vi "Main Page.vi"(8 "error in (no error)":errorcluster, 11 "Node Ptr":T2 format="%.0x") -> (0 "error out":errorcluster)   [LabVIEW 2019, in "TimingDRV System Explorer.lvlib"]
uses:
  TimingDRV System Explorer.lvlib
  <vilib>/NI VeriStand/Custom Device API/Custom Device Item Ref.ctl
  TypeDefs/Operating Mode Types.ctl
  <vilib>/NI VeriStand/Custom Device API/Custom Device API.lvlib
panel:
  in  "Select operating mode":bool
  out "Operating mode":T1=enum."Single Stepping"
  in  "Header":cluster{"Section Name":string}={"Section Name"="Custom Device Item Settings"}
  out "Name":string
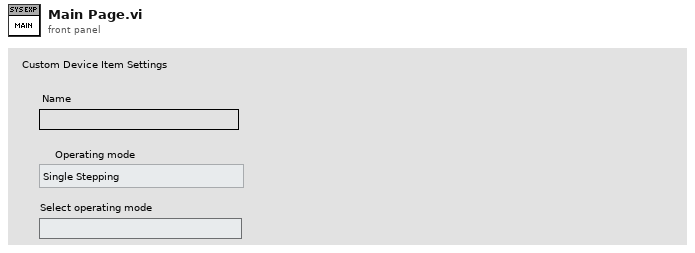
[diagram p1: front panel]
types:
  T1 = typedef "TimingDRV System Explorer.lvlib/Operating Mode Types.ctl" = enum16{"Free Running", "Single Stepping"}
  T2 = typedef "Custom Device API.lvlib/Custom Device Item Ref.ctl" = u64
  T3 = typedef "Custom Device API.lvlib/Custom Device Item Info.ctl" = cluster{"Name":string, "Is Channel":bool, "GUID":string, "Is Waveform":bool}
  T4 = typedef "Custom Device API.lvlib/Custom Device Commands.ctl" = enum16{"Default", "Item renamed", "Shutdown", "Dynamic button pressed"}
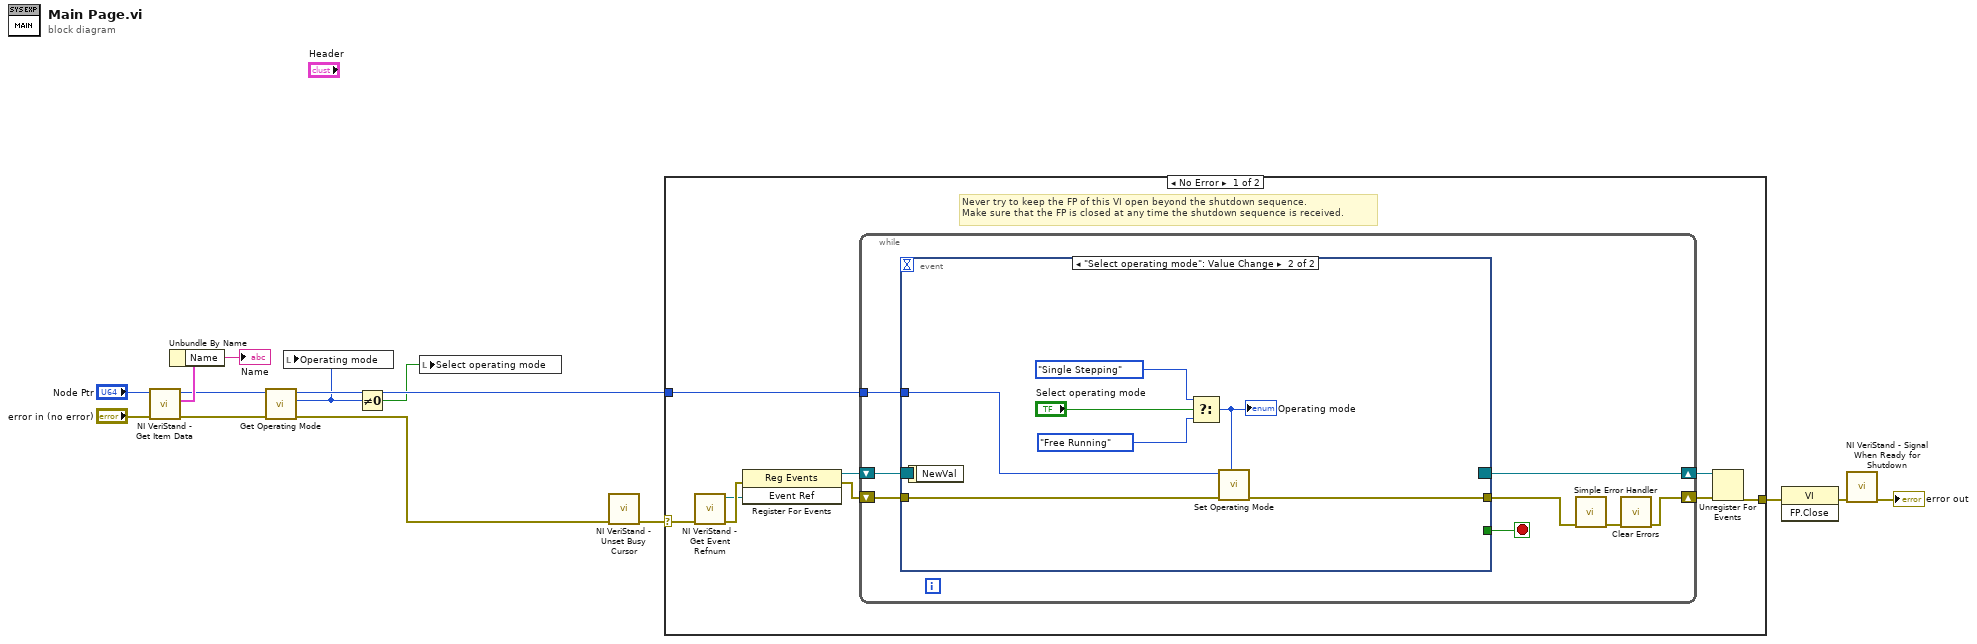
[diagram p0: block diagram]
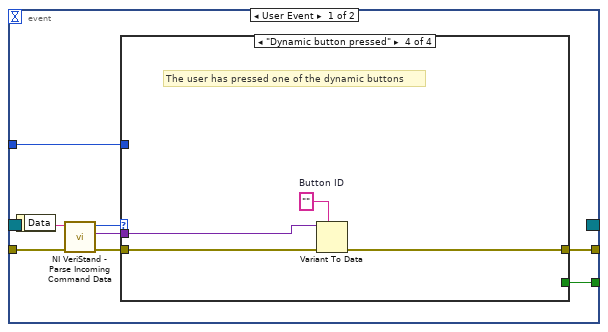
[diagram p2: hidden frame]
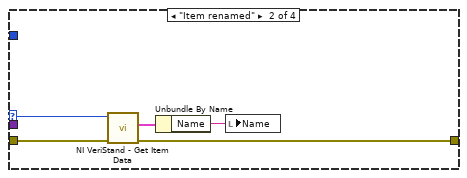
[diagram p4: hidden frame]
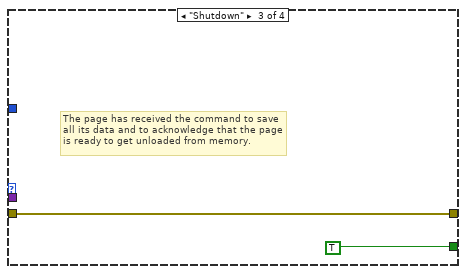
[diagram p5: hidden frame]
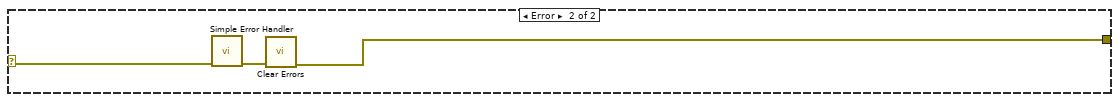
[diagram p6: hidden frame]
diagram:
  n1 = call <vilib>:"NI VeriStand - Get Item Data.vi"("error in (no error)"="error in (no error)", "Item Ref in"="Node Ptr") -> ("error out"=w5:errorcluster, "Item Info"=w8:T3, "Item Ref out"=w6:T2)  [unwired: 7 out]
  n2 = Unbundle By Name(w8) -> ("Name"=→"Name":string)
  n3 = call "Get Operating Mode.vi"("error in (no error)"=w5, "Item Ref in"=w6) -> ("error out"=w3:errorcluster, "Operating mode"=w2:T1, "Item Ref out"=w4:T2)  [unwired: 7 in]
  n4 = local write "Operating mode"(w2) -> ()
  n5 = Not Equal To 0?(x=w2) -> (x != 0?=w1:bool)
  n6 = local write "Select operating mode"(w1) -> ()
  n7 = call <vilib>:"NI VeriStand - Unset Busy Cursor.vi"("error in (no error)"=w3) -> ("error out"=w10:errorcluster)  [unwired: 10 out]
  n8 = case shown="No Error" w10 {
    selector: w10 -> [w16 w61]
    tunnel: [w20 w59] -> w14
    tunnel: w4 -> [w17 _]
    frame No Error {
      # "Never try to keep the FP of this VI open beyond the shutdown sequence.\nMake sure that the FP is closed at any time the shutdown sequence is received."
      n9 = call <vilib>:"NI VeriStand - Get Event Refnum.vi"("error in (no error)"=w16) -> ("error out"=w23:errorcluster, "Event Ref"=w19:refnum<user-event>)  [unwired: 9 out]
      n10 = register-events(error in=w23, w19) -> (reference out=w18:refnum<event-registration>, error out=w15:errorcluster)  [unwired: 1 in]
      n11 = while {
        tunnel: w17 -> [w27]
        shift-right: [w24] -> w21
        shift-left: w15 -> [w30]
        shift-right: [w31] -> w22
        shift-left: w18 -> [w29]
        stop <- w28 stop-if-true
        n12 = event shown="[1] \"Select operating mode\": Value Change" {
          selector: w29 -> [_ _]
          dyn-events: [_ _] -> w31
          timeout: _ -> [_ _]
          tunnel: w30 -> [w39 w58]
          tunnel: [w35 _] -> w28
          tunnel: [w34 w52] -> w26
          tunnel: w27 -> [w33 w54]
          event User Event {
            n13 = event-data() -> ("Data"=w38:string)  [unwired: 1 out]
            n14 = call <vilib>:"NI VeriStand - Parse Incoming Command Data.vi"("error in (no error)"=w39, "Incoming data"=w38) -> ("error out"=w37:errorcluster, "Outgoing data"=w32:variant, "Action"=w36:T4)  [unwired: 7 out]
            n15 = case shown="\"Dynamic button pressed\"" w36 {
              tunnel: w37 -> [w40 w45 w46 w49]
              tunnel: [_ _ TRUE _] -> w35
              tunnel: [w40 w42 w46 w50] -> w34
              tunnel: w33 -> [_ w44 _ _]
              tunnel: w32 -> [_ _ _ w48]
              frame "Default", Default {
              }
              frame "Item renamed" {
                n16 = call <vilib>:"NI VeriStand - Get Item Data.vi"("error in (no error)"=w45, "Item Ref in"=w44) -> ("error out"=w42:errorcluster, "Item Info"=w43:T3)  [unwired: 8 out]
                n17 = Unbundle By Name(w43) -> ("Name"=w41:string)
                n18 = local write "Name"(w41) -> ()
              }
              frame "Shutdown" {
                # "The page has received the command to save all its data and to acknowledge that the page is ready to get unloaded from memory."
              }
              frame "Dynamic button pressed" {
                w51 = ""  # Button ID
                # "The user has pressed one of the dynamic buttons"
                n19 = Variant To Data(error in=w49, type=w51, Variant=w48) -> (error out=w50:errorcluster)  [unwired: 1 out]
              }
            }
          }
          event "Select operating mode": Value Change {
            n20 = event-data() -> ()  [unwired: 2 out]
            n21 = Select(t=Operating_Mode_Types."Single Stepping" ("Operating mode"), s="Select operating mode", f=Operating_Mode_Types."Free Running" ("Operating mode")) -> (s? t:f=w53:T1)
            "Operating mode" <- w53
            n22 = call "Set Operating Mode.vi"("Operating mode"=w53, "error in (no error)"=w58, "CD Ref in"=w54) -> ("error out"=w52:errorcluster)  [unwired: 7 in, 1 out]
          }
        }
        n23 = call <vilib>:"Simple Error Handler.vi"("error in (no error)"=w26) -> ("error out"=w25:errorcluster)  [unwired: 1 in, 7 out]
        n24 = call <vilib>:"Clear Errors.vi"("error in (no error)"=w25) -> ("error out"=w24:errorcluster)  [unwired: 1 in, 5 out]
      }
      n25 = Unregister For Events(event registration refnum=w22, error in=w21) -> (error out=w20:errorcluster)
    }
    frame Error {
      n26 = call <vilib>:"Simple Error Handler.vi"("error in (no error)"=w61) -> ("error out"=w60:errorcluster)  [unwired: 1 in, 7 out]
      n27 = call <vilib>:"Clear Errors.vi"("error in (no error)"=w60) -> ("error out"=w59:errorcluster)  [unwired: 1 in, 5 out]
    }
  }
  n28 = invoke class="VI" method="FP.Close"(error in=w14) -> (error out=w13:errorcluster)  [unwired: 2 in, 2 out]
  n29 = call <vilib>:"NI VeriStand - Signal When Ready for Shutdown.vi"("error in (no error)"=w13) -> ("error out"=→"error out":errorcluster)  [unwired: 10 out]
